vi "Update Inst Config.vi"(8 "error in (no error)":errorcluster, 11 "Data In":string[](array[string])) -> (0 "error out":errorcluster, 3 "Inst Config":T1={"Connection"={"Ref"=variant, "Serial"={"Baud Rate"=9600, "Parity"=0, "Data Bits"=8, "Flow Control"=4}}, "Ouput Imp"={"User-Defined Impedance (50 Ohms)"=50.0, "Impedance (0: 50 Ohms)"=0}} {"Connection"."Serial"."Baud Rate" items=["300"=300, "600"=600, "1200"=1200, "2400"=2400, "4800"=4800, "9600"=9600, "19200"=19200]; "Connection"."Serial"."Parity" items=["None", "Odd", "Even", "Mark", "Space"]; "Connection"."Serial"."Data Bits" items=["7"=7, "8"=8]; "Connection"."Serial"."Flow Control" items=["None", "XON/XOFF", "RTS/CTS", "XON/XOFF & RTS/CTS", "DTR/DSR", "XON/XOFF & DTR/DSR"]; "Ouput Imp"."Impedance (0: 50 Ohms)" items=["50 Ohms", "High Impedance", "User Defined"]})   [LabVIEW 2016, in "Func Generator.lvlib"]
uses:
  Func Generator.lvlib
  Inst Config Parameter.ctl
panel:
  in  "Flow Control":u16(ring)=4 items=["None", "XON/XOFF", "RTS/CTS", "XON/XOFF & RTS/CTS", "DTR/DSR", "XON/XOFF & DTR/DSR"]
  in  "Parity":u16(ring) items=["None", "Odd", "Even", "Mark", "Space"]
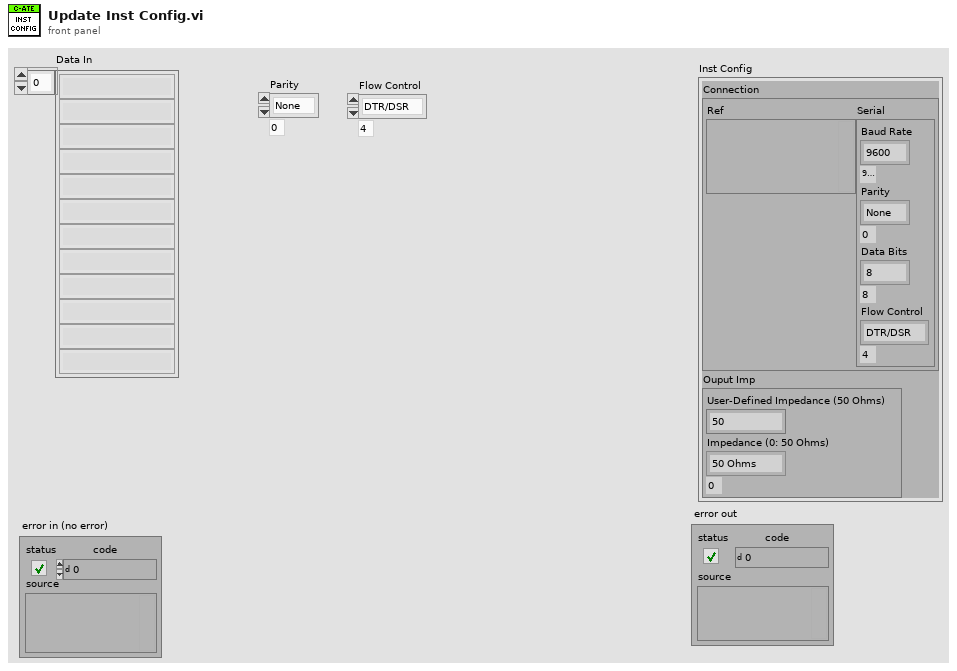
[diagram p1: front panel]
types:
  T1 = typedef "Func Generator.lvlib/Inst Config Parameter.ctl" = cluster{"Connection":cluster{"Ref":variant, "Serial":cluster{"Baud Rate":u32, "Parity":u16, "Data Bits":u16, "Flow Control":u16}}, "Ouput Imp":cluster{"User-Defined Impedance (50 Ohms)":dbl, "Impedance (0: 50 Ohms)":u16}}
  T2 = typedef "LVStringsAndValuesArrayTypeDef_U16.ctl" = cluster{"String":string, "Value":u16}[]
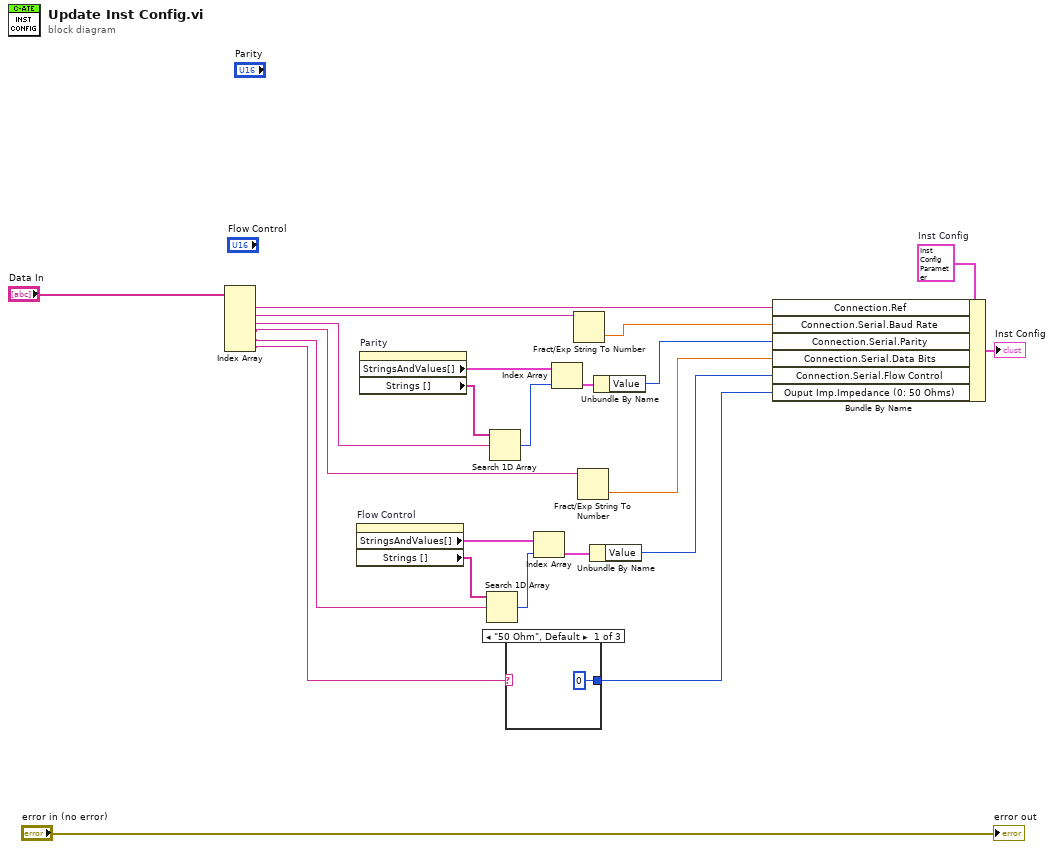
[diagram p0: block diagram]
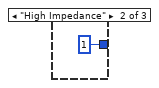
[diagram p2: hidden frame]
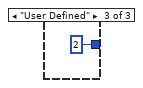
[diagram p3: hidden frame]
diagram:
  w21 = T1 {"Connection"={"Ref"=variant, "Serial"={"Baud Rate"=9600, "Parity"=0, "Data Bits"=8, "Flow Control"=4}}, "Ouput Imp"={"User-Defined Impedance (50 Ohms)"=50.0, "Impedance (0: 50 Ohms)"=0}}  # Inst Config
  n1 = Index Array(array="Data In") -> (element #1=w19:string, element #2=w18:string, element #3=w11:string, element #4=w10:string, element #5=w6:string, element #6=w2:string)  [unwired: 6 in]
  n2 = property on="Flow Control" class="Ring (strict)"() -> ("StringsAndValues[]"=w8:T2, "Strings []"=w7:string[])  [unwired: 2 in, 2 out]
  n3 = property on="Parity" class="Ring (strict)"() -> ("StringsAndValues[]"=w15:T2, "Strings []"=w16:string[])  [unwired: 2 in, 2 out]
  n4 = Search 1D Array(1D array=w7, element=w6) -> (index of element=w5:i32)  [unwired: 1 in]
  n5 = Search 1D Array(1D array=w16, element=w11) -> (index of element=w14:i32)  [unwired: 1 in]
  n6 = case shown="\"50 Ohm\", Default" w2 {
    tunnel: [u16 0 ("Ouput Imp.Impedance (0: 50 Ohms)") u16 1 ("Ouput Imp.Impedance (0: 50 Ohms)") u16 2 ("Ouput Imp.Impedance (0: 50 Ohms)")] -> w1
    frame "50 Ohm", Default {
    }
    frame "High Impedance" {
    }
    frame "User Defined" {
    }
  }
  n7 = Index Array(array=w8, index=w5) -> (element=w4:cluster{"String":string, "Value":u16})
  n8 = Index Array(array=w15, index=w14) -> (element=w13:cluster{"String":string, "Value":u16})
  n9 = Fract/Exp String To Number(string=w18) -> (number=w17:dbl)  [unwired: 3 in, 1 out]
  n10 = Fract/Exp String To Number(string=w10) -> (number=w9:dbl)  [unwired: 3 in, 1 out]
  n11 = Unbundle By Name(w4) -> ("Value"=w3:u16)
  n12 = Unbundle By Name(w13) -> ("Value"=w12:u16)
  n13 = Bundle By Name(cluster=w21, "Connection.Ref"=w19, "Connection.Serial.Baud Rate"=w17, "Connection.Serial.Parity"=w12, "Connection.Serial.Data Bits"=w9, "Connection.Serial.Flow Control"=w3, "Ouput Imp.Impedance (0: 50 Ohms)"=w1) -> (→"Inst Config":T1)
  "error out" <- "error in (no error)"
